vi "Destroy Client.vi"(8 "error in":errorcluster) -> (0 "error out":errorcluster)   [LabVIEW 2021, in "NI Discovery V1 Client.lvlib"]
uses:
  NI Discovery V1 Client.lvlib
  TypeDefs/gRPC Client Cache FGV Action.ctl
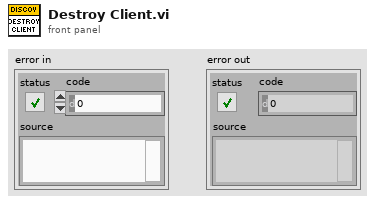
[diagram p1: front panel]
types:
  T1 = typedef "NI Discovery V1 Client.lvlib/gRPC Client Cache FGV Action.ctl" = enum16{"Get Client", "Recreate Client", "Destroy Client", "Update ClusterId"}
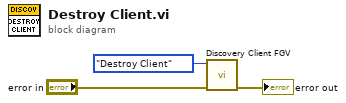
[diagram p0: block diagram]
diagram:
  n1 = call "Discovery Client FGV.vi"("error in"="error in", "action"=gRPC_Client_Cache_FGV_Action."Destroy Client") -> ("error out"=→"error out":errorcluster)  [unwired: 6 in, 3 out]
